vi "Load_All_Transconductance_2D angles_use this one.vi"() -> ()   [LabVIEW 2016]
panel:
  out "peak diff large":T1(graph)=[{"Vfast"=[182.012, 179.504, 177.006, 174.535, 172.007, 169.511, 167.008, 164.51, 162.009, 159.505, 157.011], "Decimated Array"=[106.1367318836291, 107.9166309553778, 108.03439594283006, 108.95926450557812, 110.67695734065168, 109.44953149085208, 110.59557079304213, 111.94164984286797, 109.40881307605187, 107.22139343937062, 107.79343273045154]}, {"Vfast"=[182.012, 179.504, 177.006, 174.535, 172.007, 169.511, 167.008, 164.51, 162.009, 159.505, 157.011], "Decimated Array"=[105.14063187449949, 107.41646243515345, 107.21220328119014, 109.8178288365934, 111.23346658775407, 110.90399917792041, 110.95957413889423, 110.9751389109858, 109.02606988396329, 107.72291905671233, 105.89277234820085]}, {"Vfast"=[182.012, 179.504, 177.006, 174.535, 172.007, 169.511, 167.008, 164.51, 162.009, 159.505, 157.011], "Decimated Array"=[106.16015627089425, 107.95596762325218, 107.6583045730433, 110.98911313331146, 109.94558691039819, 111.03790978769842, 111.31345664920616, 111.74994430125929, 109.91182303380046, 108.5050531124582, 106.85785120675709]}, {"Vfast"=[182.012, 179.504, 177.006, 174.535, 172.007, 169.511, 167.008, 164.51, 162.009, 159.505, 157.011], "Decimated Array"=[107.20587316206647, 108.05227816279267, 106.49228012360808, 109.25183588381492, 109.9103591250815, 108.96767176290706, 111.22713058561078, 111.82656269636027, 108.69558441646404, 107.92630267985967, 106.29740488437943]}, {"Vfast"=[182.012, 179.504, 177.006, 174.535, 172.007, 169.511, 167.008, 164.51, 162.009, 159.505, 157.011], "Decimated Array"=[105.14473500879657, 109.01254695226427, 110.08871345320455, 109.31692443429532, 109.93396377276349, 109.03252922039067, 111.45567713682095, 109.94658582480304, 109.05288659218584, 107.32906660669974, 106.53504425061402]}, {"Vfast"=[182.012, 179.504, 177.006, 174.535, 172.007, 169.511, 167.008, 164.51, 162.009, 159.505, 157.011], "Decimated Array"=[105.2880346854731, 106.69565142870721, 110.1246624621377, 109.77721530893652, 110.08443910203746, 110.06271173431094, 110.35514216658441, 111.80901475091426, 109.04382568493875, 106.82278931215859, 106.04892396437907]}, {"Vfast"=[182.012, 179.504, 177.006, 174.535, 172.007, 169.511, 167.008, 164.51, 162.009, 159.505, 157.011], "Decimated Array"=[106.72911315514773, 106.93463737892725, 109.21719703822447, 110.13824399378325, 109.08707239851142, 109.51635999510242, 110.75653832860385, 111.13863025041724, 109.8978999144289, 107.81607740080258, 104.98521261437102]}, {"Vfast"=[182.012, 179.504, 177.006, 174.535, 172.007, 169.511, 167.008, 164.51, 162.009, 159.505, 157.011], "Decimated Array"=[106.80512670799465, 106.09499848275524, 108.59345782796484, 111.07213572882122, 111.05363353698229, 109.97447722536103, 111.95362061630311, 112.0573743847792, 109.54990665167563, 108.91459550205761, 103.96113162752582]}, {"Vfast"=[182.012, 179.504, 177.006, 174.535, 172.007, 169.511, 167.008, 164.51, 162.009, 159.505, 157.011], "Decimated Array"=[104.09691032567451, 106.58955949054447, 109.85173826113416, 109.85010031222419, 110.19174517224519, 110.98416054822326, 111.11132375674154, 111.03774101973798, 108.06195790942536, 107.48717576844453, 104.32959579304895]}, {"Vfast"=[182.012, 179.504, 177.006, 174.535, 172.007, 169.511, 167.008, 164.51, 162.009, 159.505, 157.011], "Decimated Array"=[105.4658044990251, 105.74662923765885, 109.7660935832223, 110.90835697296129, 111.1645265426047, 110.9223147774517, 110.75222743652645, 110.08793310583437, 108.15329429958669, 106.6561368020513, 105.29878368846795]}, {"Vfast"=[182.012, 179.504, 177.006, 174.535, 172.007, 169.511, 167.008, 164.51, 162.009, 159.505, 157.011], "Decimated Array"=[104.71173984282939, 106.04073481441341, 108.88654524231296, 110.02841877426988, 110.72449573620023, 110.07415564747015, 111.2712095961179, 110.87580773627934, 111.15970574227836, 107.84436875778428, 105.02397493400468]}, {"Vfast"=[182.012, 179.504, 177.006, 174.535, 172.007, 169.511, 167.008, 164.51, 162.009, 159.505, 157.011], "Decimated Array"=[103.06846731187167, 106.89645794027464, 111.60777545833645, 111.22600855781286, 109.15261842050231, 110.95233315826488, 110.34706056930082, 111.07802963390537, 109.39849805700513, 107.00240295220092, 104.7204338369038]}, {"Vfast"=[182.012, 179.504, 177.006, 174.535, 172.007, 169.511, 167.008, 164.51, 162.009, 159.505, 157.011], "Decimated Array"=[103.2976624060164, 106.99558877972262, 110.34188694884759, 110.10205985628787, 110.68096476308085, 109.2627256399542, 112.01875972082743, 111.90171808566129, 107.34991285375341, 105.21978562040852, 104.08956766104328]}]
  out "large angles":dbl[][](array[numeric])
  out "peak diff small":T1(graph)=[{"Vfast"=[152.611, 154.521, 157.019, 159.159, 161.982, 164.502, 166.904, 169.371, 171.997, 174.501, 176.701, 179.487, 181.998], "Decimated Array"=[106.1367318836291, 105.14063187449949, 106.16015627089425, 107.20587316206647, 105.14473500879657, 105.2880346854731, 106.72911315514773, 106.80512670799465, 104.09691032567451, 105.4658044990251, 104.71173984282939, 103.06846731187167, 103.2976624060164]}, {"Vfast"=[182.007, 179.827, 176.956, 174.514, 172.174, 169.502, 167.252, 164.512, 162.068, 159.491, 157.22, 154.749, 152.204], "Decimated Array"=[106.99558877972262, 106.89645794027464, 106.04073481441341, 105.74662923765885, 106.58955949054447, 106.09499848275524, 106.93463737892725, 106.69565142870721, 109.01254695226427, 108.05227816279267, 107.95596762325218, 107.41646243515345, 107.9166309553778]}, {"Vfast"=[151.995, 154.396, 156.992, 159.309, 161.993, 164.281, 166.816, 169.292, 172.022, 174.29, 176.983, 178.925, 181.965], "Decimated Array"=[108.03439594283006, 107.21220328119014, 107.6583045730433, 106.49228012360808, 110.08871345320455, 110.1246624621377, 109.21719703822447, 108.59345782796484, 109.85173826113416, 109.7660935832223, 108.88654524231296, 111.60777545833645, 110.34188694884759]}, {"Vfast"=[181.998, 179.507, 177.004, 174.498, 172.23, 169.474, 167.212, 164.881, 162.178, 159.922, 157.024, 154.742, 152.001], "Decimated Array"=[110.10205985628787, 111.22600855781286, 110.02841877426988, 110.90835697296129, 109.85010031222419, 111.07213572882122, 110.13824399378325, 109.77721530893652, 109.31692443429532, 109.25183588381492, 110.98911313331146, 109.8178288365934, 108.95926450557812]}, {"Vfast"=[151.993, 154.261, 156.807, 159.134, 161.987, 164.278, 167.0, 169.414, 171.78, 174.418, 176.847, 179.499, 181.743], "Decimated Array"=[110.67695734065168, 111.23346658775407, 109.94558691039819, 109.9103591250815, 109.93396377276349, 110.08443910203746, 109.08707239851142, 111.05363353698229, 110.19174517224519, 111.1645265426047, 110.72449573620023, 109.15261842050231, 110.68096476308085]}, {"Vfast"=[182.003, 179.724, 177.288, 174.502, 172.408, 169.784, 167.224, 164.787, 162.208, 159.929, 157.013, 154.684, 152.303], "Decimated Array"=[109.2627256399542, 110.95233315826488, 110.07415564747015, 110.9223147774517, 110.98416054822326, 109.97447722536103, 109.51635999510242, 110.06271173431094, 109.03252922039067, 108.96767176290706, 111.03790978769842, 110.90399917792041, 109.44953149085208]}, {"Vfast"=[151.975, 154.281, 156.97, 159.168, 161.748, 164.403, 166.864, 169.32, 171.787, 174.225, 176.792, 179.243, 181.729], "Decimated Array"=[110.59557079304213, 110.95957413889423, 111.31345664920616, 111.22713058561078, 111.45567713682095, 110.35514216658441, 110.75653832860385, 111.95362061630311, 111.11132375674154, 110.75222743652645, 111.2712095961179, 110.34706056930082, 112.01875972082743]}, {"Vfast"=[182.003, 179.494, 177.325, 174.834, 172.15, 169.73, 167.039, 164.719, 161.997, 159.871, 157.373, 154.751, 152.344], "Decimated Array"=[111.90171808566129, 111.07802963390537, 110.87580773627934, 110.08793310583437, 111.03774101973798, 112.0573743847792, 111.13863025041724, 111.80901475091426, 109.94658582480304, 111.82656269636027, 111.74994430125929, 110.9751389109858, 111.94164984286797]}, {"Vfast"=[152.344, 154.493, 156.98, 159.478, 161.958, 164.262, 166.85, 169.347, 172.005, 174.21, 177.009, 179.386, 181.876], "Decimated Array"=[109.40881307605187, 109.02606988396329, 109.91182303380046, 108.69558441646404, 109.05288659218584, 109.04382568493875, 109.8978999144289, 109.54990665167563, 108.06195790942536, 108.15329429958669, 111.15970574227836, 109.39849805700513, 107.34991285375341]}, {"Vfast"=[182.002, 179.505, 177.231, 174.768, 172.352, 169.744, 167.018, 164.748, 162.011, 159.877, 157.405, 154.737, 152.281], "Decimated Array"=[105.21978562040852, 107.00240295220092, 107.84436875778428, 106.6561368020513, 107.48717576844453, 108.91459550205761, 107.81607740080258, 106.82278931215859, 107.32906660669974, 107.92630267985967, 108.5050531124582, 107.72291905671233, 107.22139343937062]}, {"Vfast"=[152.002, 154.502, 156.649, 159.501, 161.992, 164.318, 166.897, 169.419, 171.88, 174.293, 176.902, 179.179, 182.022], "Decimated Array"=[107.79343273045154, 105.89277234820085, 106.85785120675709, 106.29740488437943, 106.53504425061402, 106.04892396437907, 104.98521261437102, 103.96113162752582, 104.32959579304895, 105.29878368846795, 105.02397493400468, 104.7204338369038, 104.08956766104328]}]
  out "Intensity Graph 15":dbl[][](graph)
  in  "index (page)":i32=3
  out "Intensity Graph 14":dbl[][](graph)
  out "small angles":dbl[][](array[numeric])
  in  "read data from file?":bool
  out "All Folders":path[](array[path])=[path "P:/expt/Leiden MNK/SA02836H.20170110/40/40 - Sweep axis 1,2 - 0", path "P:/expt/Leiden MNK/SA02836H.20170110/40/40 - Sweep axis 1,2 - 1", path "P:/expt/Leiden MNK/SA02836H.20170110/40/40 - Sweep axis 1,2 - 2", path "P:/expt/Leiden MNK/SA02836H.20170110/40/40 - Sweep axis 1,2 - 3", path "P:/expt/Leiden MNK/SA02836H.20170110/40/40 - Sweep axis 1,2 - 4", path "P:/expt/Leiden MNK/SA02836H.20170110/40/40 - Sweep axis 1,2 - 5", path "P:/expt/Leiden MNK/SA02836H.20170110/40/40 - Sweep axis 1,2 - 6", path "P:/expt/Leiden MNK/SA02836H.20170110/40/40 - Sweep axis 1,2 - 7", path "P:/expt/Leiden MNK/SA02836H.20170110/40/40 - Sweep axis 1,2 - 8", path "P:/expt/Leiden MNK/SA02836H.20170110/40/40 - Sweep axis 1,2 - 9", path "P:/expt/Leiden MNK/SA02836H.20170110/40/x40 - Sweep axis 1,2 - 10"]
  out "Numeric":i32=10
  out "Array":i32[][](array[numeric])
  in  "Array 2":path[](array[path])=[path "P:/expt/Leiden MNK/SA02836H.20170110/40"]
  out "Intensity Graph 12":dbl[][][](array[numeric])
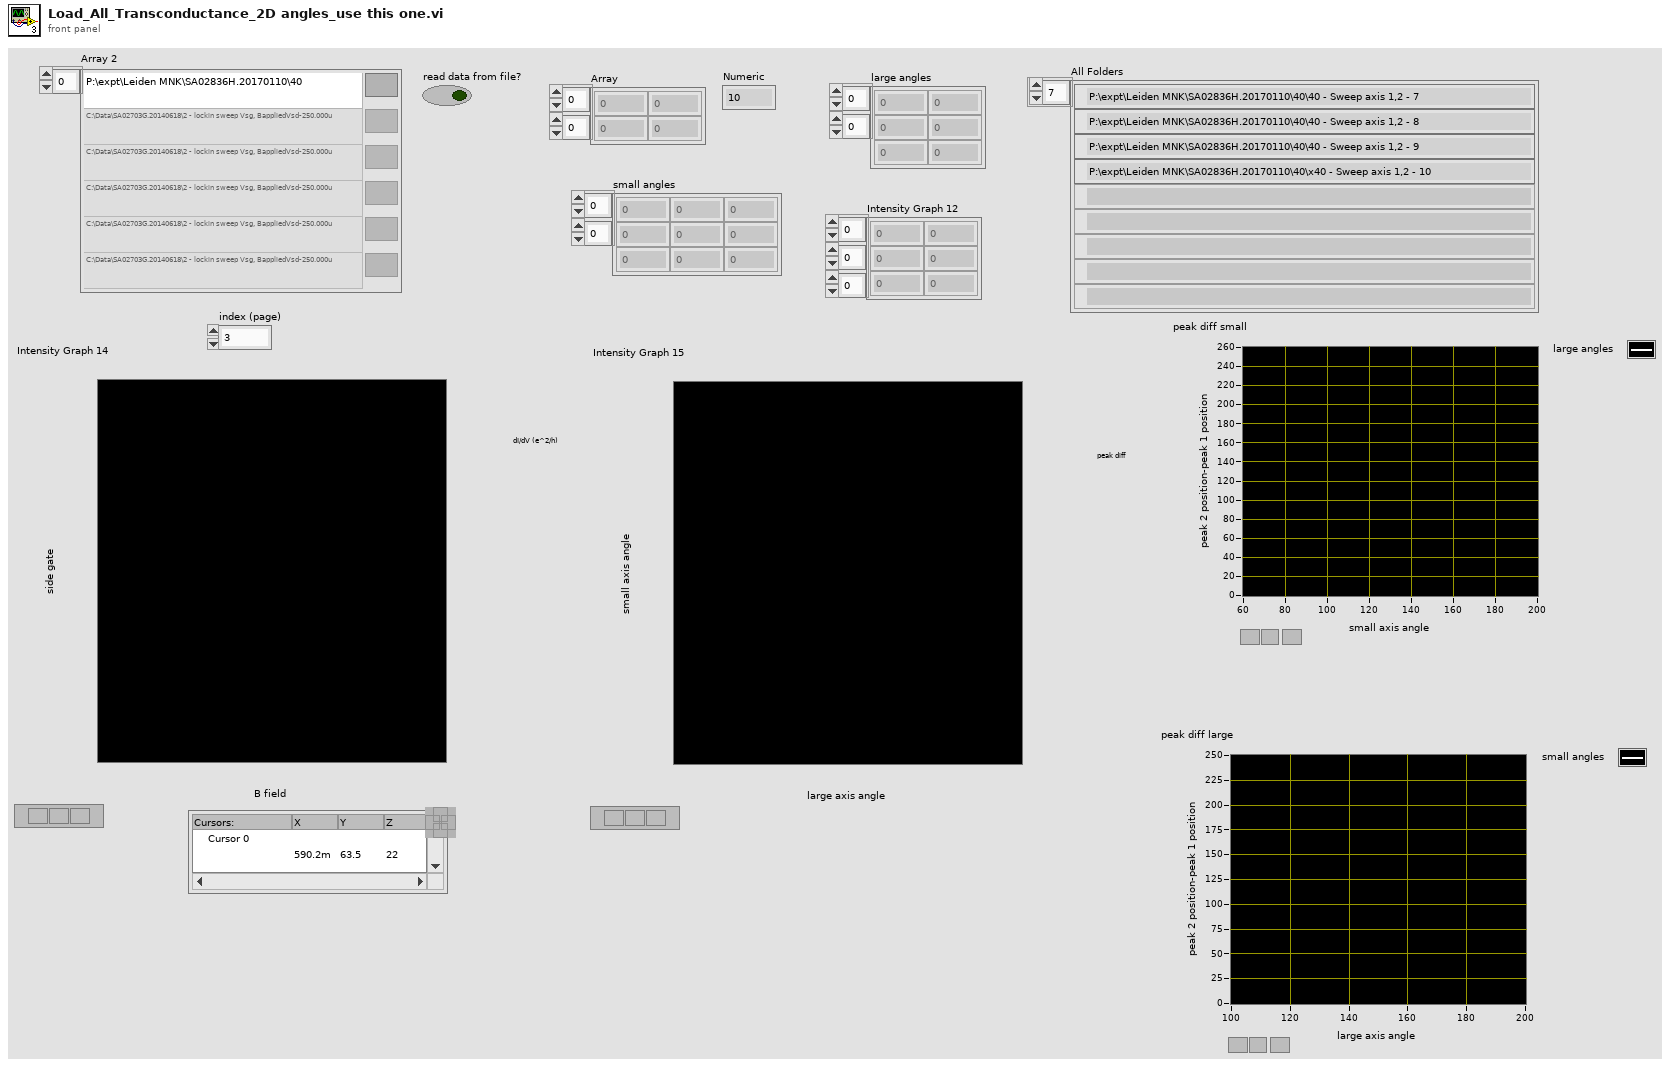
[diagram p1: front panel]
types:
  T1 = cluster{"Vfast":dbl[], "Decimated Array":dbl[]}[]
  T2 = cluster{"N1":dbl, "N2":dbl, "N3":dbl, "N4":dbl}[]
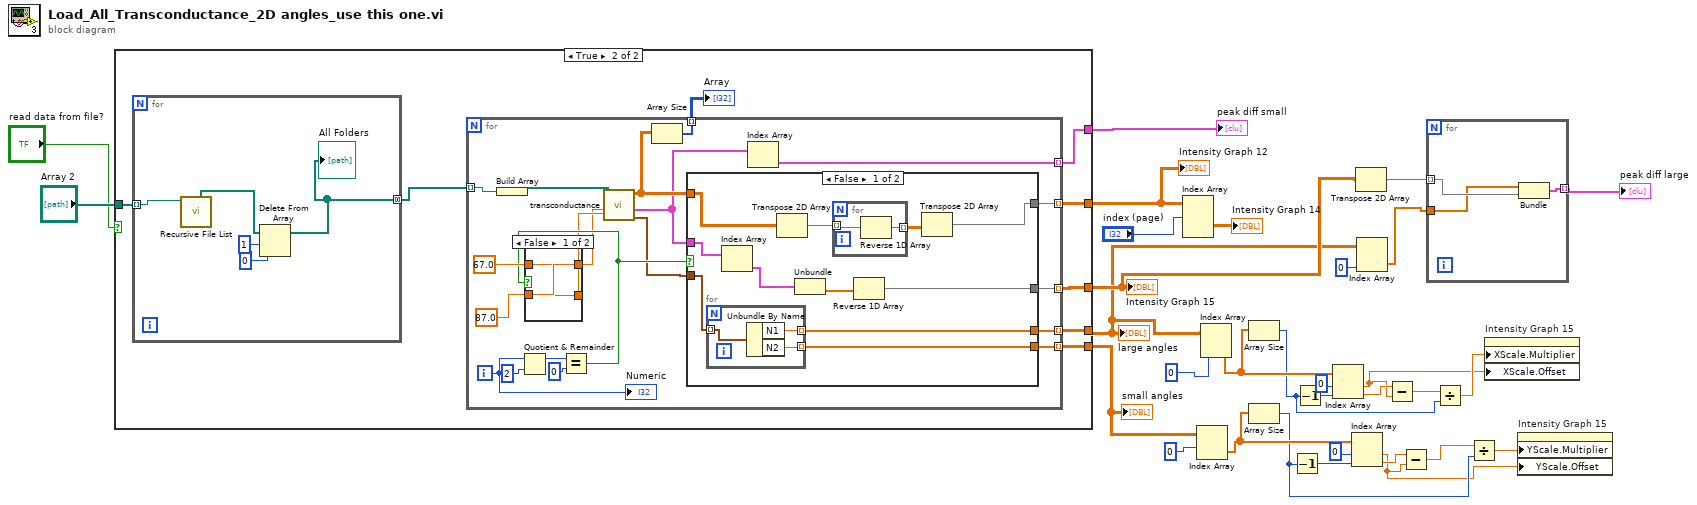
[diagram p0: block diagram]
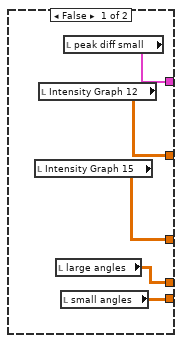
[diagram p2: hidden frame]
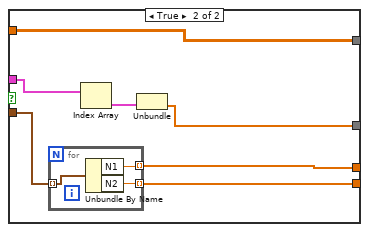
[diagram p3: hidden frame]
diagram:
  n1 = case shown="True" "read data from file?" {
    tunnel: "Array 2" -> [_ w44]
    tunnel: [w36 w42] -> w28
    tunnel: [w35 w40] -> w25
    tunnel: [w34 w39] -> w5
    tunnel: [w33 w38] -> w26
    tunnel: [w32 w37] -> w1
    frame False {
      n2 = local read "Intensity Graph 15"() -> (w34:dbl[][])
      n3 = local read "Intensity Graph 12"() -> (w36:dbl[][][])
      n4 = local read "large angles"() -> (w32:dbl[][])
      n5 = local read "small angles"() -> (w35:dbl[][])
      n6 = local read "peak diff small"() -> (w33:T1)
    }
    frame True {
      n7 = for {
        tunnel: w44 -> [w99] mode=indexing
        tunnel: [w95] -> w43 mode=concatenating
        n8 = call <vilib>:"Recursive File List.vi"("Folder Path"=w99) -> ("All Folders"=w98:path[])  [unwired: 6 in, 4 out]
        n9 = Delete From Array(array=w98, length=1, index=0) -> (array with subset deleted=w95:path[])  [unwired: 1 out]
        "All Folders" <- w95
      }
      n10 = for {
        tunnel: w43 -> [w64] mode=indexing
        tunnel: [w60] -> w42 mode=indexing
        tunnel: [w53] -> w41 mode=indexing
        tunnel: [w51] -> w40 mode=indexing
        tunnel: [w47] -> w39 mode=indexing
        tunnel: [w50] -> w38 mode=indexing
        tunnel: [w49] -> w37 mode=indexing
        i -> [w59]
        n11 = Build Array(w64) -> (w63:path[])
        n12 = Quotient & Remainder(x=w59, y=2) -> (x-y*floor(x/y)=w57:i32)  [unwired: 1 out]
        n13 = Equal?(x=w57, y=0) -> (x = y?=w55:bool)
        n14 = call "transconductance.vi"("New Files to Process"=w63) -> ("N Array"=w52:T2, "peak diff"=w48:T1, "Intensity Graph 12"=w54:dbl[][], "B max"=w46:dbl, "B min"=w45:dbl)  [unwired: 5 in, 1 out]
        n15 = case shown="False" w55 {
          tunnel: 67.0 ("B min") -> [w91 w94]
          tunnel: w45 -> [w92 w94]
          tunnel: 87.0 ("B max") -> [w92 w93]
          tunnel: w46 -> [w91 w93]
          frame False {
          }
          frame True {
          }
        }
        n16 = Array Size(array=w54) -> (size(s)=w53:i32[])
        n17 = case shown="False" w55 {
          tunnel: w54 -> [w75 w87]
          tunnel: [w72 w87] -> w60
          tunnel: w52 -> [w71 w86]
          tunnel: [w70 w85] -> w51
          tunnel: [w69 w84] -> w49
          tunnel: w48 -> [w68 w83]
          tunnel: [w65 w81] -> w47
          frame False {
            n18 = for {
              tunnel: w71 -> [w78] mode=indexing
              tunnel: [w77] -> w69 mode=indexing
              tunnel: [w76] -> w70 mode=indexing
              n19 = Unbundle By Name(w78) -> ("N1"=w77:dbl, "N2"=w76:dbl)
            }
            n20 = Index Array(array=w68) -> (element=w67:cluster{"Vfast":dbl[], "Decimated Array":dbl[]})  [unwired: 1 in]
            n21 = Transpose 2D Array(2D array=w75) -> (transposed array=w74:dbl[][])
            n22 = Unbundle(w67) -> ("Decimated Array"=w66:dbl[])  [unwired: 1 out]
            n23 = for {
              tunnel: w74 -> [w80] mode=indexing
              tunnel: [w79] -> w73 mode=indexing
              n24 = Reverse 1D Array(array=w80) -> (reversed array=w79:dbl[])
            }
            n25 = Reverse 1D Array(array=w66) -> (reversed array=w65:dbl[])
            n26 = Transpose 2D Array(2D array=w73) -> (transposed array=w72:dbl[][])
          }
          frame True {
            n27 = for {
              tunnel: w86 -> [w90] mode=indexing
              tunnel: [w89] -> w85 mode=indexing
              tunnel: [w88] -> w84 mode=indexing
              n28 = Unbundle By Name(w90) -> ("N1"=w88:dbl, "N2"=w89:dbl)
            }
            n29 = Index Array(array=w83) -> (element=w82:cluster{"Vfast":dbl[], "Decimated Array":dbl[]})  [unwired: 1 in]
            n30 = Unbundle(w82) -> ("Decimated Array"=w81:dbl[])  [unwired: 1 out]
          }
        }
        n31 = Index Array(array=w48) -> (element=w50:cluster{"Vfast":dbl[], "Decimated Array":dbl[]})  [unwired: 1 in]
        "Numeric" <- w59
      }
      "Array" <- w41
    }
  }
  "Intensity Graph 12" <- w28
  "small angles" <- w25
  "Intensity Graph 15" <- w5
  "peak diff small" <- w26
  "large angles" <- w1
  n32 = Index Array(array=w28, index (dim 0)="index (page)") -> (element=→"Intensity Graph 14":dbl[][])  [unwired: 2 in]
  n33 = Index Array(array=w25, index (row)=0) -> (element=w20:dbl[])  [unwired: 1 in]
  n34 = Index Array(array=w1, index (col)=0 ("index (row)")) -> (element=w22:dbl[])  [unwired: 1 in]
  n35 = Array Size(array=w22) -> (size(s)=w16:i32)
  n36 = Array Size(array=w20) -> (size(s)=w15:i32)
  n37 = Decrement(x=w15) -> (x-1=w19:i32)
  n38 = Decrement(x=w16) -> (x-1=w17:i32)
  n39 = Index Array(array=w22, index #1=0 ("index (row)"), index #2=w17) -> (element #1=w7:dbl, element #2=w8:dbl)
  n40 = Index Array(array=w20, index #1=0 ("index (row)"), index #2=w19) -> (element #1=w9:dbl, element #2=w10:dbl)
  n41 = Transpose 2D Array(2D array=w5) -> (transposed array=w6:dbl[][])
  n42 = Index Array(array=w1, index (col)=0 ("disabled index (col)")) -> (element=w3:dbl[])  [unwired: 1 in]
  n43 = Subtract(x=w8, y=w7) -> (x-y=w12:dbl)
  n44 = Subtract(x=w10, y=w9) -> (x-y=w11:dbl)
  n45 = for {
    tunnel: w6 -> [w101] mode=indexing
    tunnel: w3 -> [w100]
    tunnel: [w102] -> w2 mode=indexing
    n46 = Bundle("large angles"=w100, w101) -> (w102:cluster{"large angles":dbl[], dbl[]})  [unwired: 1 in]
  }
  "peak diff large" <- w2
  n47 = Divide(x=w12, y=w16) -> (x/y=w13:dbl)
  n48 = Divide(x=w11, y=w15) -> (x/y=w14:dbl)
  n49 = property on="Intensity Graph 15" class="IntGraph (strict)"("XScale.Multiplier"=w13, "XScale.Offset"=w7) -> ()  [unwired: 2 in, 2 out]
  n50 = property on="Intensity Graph 15" class="IntGraph (strict)"("YScale.Multiplier"=w14, "YScale.Offset"=w9) -> ()  [unwired: 2 in, 2 out]
